vi "cost.vi"(8 "error in (no error)":errorcluster, 11 "HouseBlend in":refnum<class "HouseBlend.lvclass">) -> (0 "error out":errorcluster, 2 "Cost":dbl, 3 "HouseBlend out":refnum<class "HouseBlend.lvclass">)   [LabVIEW 2013, in "HouseBlend.lvclass"]
uses:
  HouseBlend.lvclass
  Beverage/Beverage.lvclass
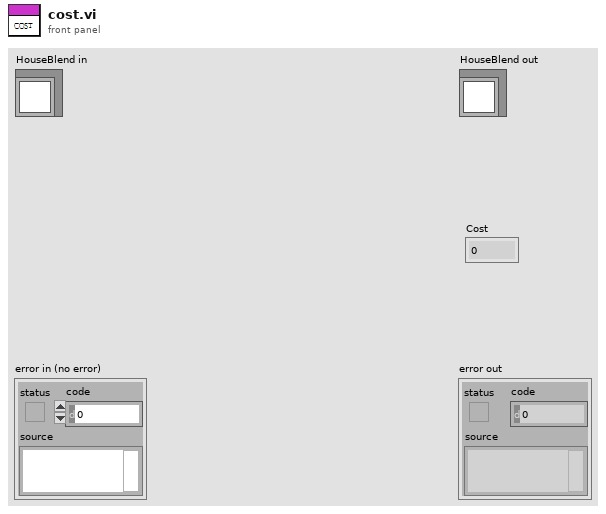
[diagram p1: front panel]
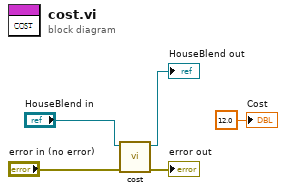
[diagram p0: block diagram]
diagram:
  n1 = call-parent "cost.vi"("error in (no error)"="error in (no error)", "Beverage in"="HouseBlend in") -> ("error out"=→"error out":errorcluster, "Beverage out"=→"HouseBlend out":refnum<class "HouseBlend.lvclass">)  [unwired: 7 in, 1 out]
  "Cost" <- 12.0 ("Cost")
